vi "ChoosePass.vi"(6 "OffensivePlay":T1, 8 "error in (no error)":errorcluster, 9 "Stk/2ndStk":enum16{"Striker", "2ndStriker"}(ring), 10 "Game":refnum<class "Game.lvclass">, 11 "Play in":refnum<class "Play.lvclass">) -> (0 "error out":errorcluster, 2 "Factor Pass":dbl, 3 "Play out":refnum<class "Play.lvclass">)   [LabVIEW 2023, in "Play.lvclass"]
uses:
  Play.lvclass
  Game_class/Game.lvclass
  Team_class/OffensivePlay.ctl
  Robot_class/roles.ctl
  Utilities_class/Utilities.lvclass
  Game_class/Game.lvclass/Game.ctl
  Team_class/Team.lvclass/Team.ctl
  Object_class/Object.lvclass/Object.ctl
  Robot_class/Robot.lvclass/Robot.ctl
  Referee_class/Referee.lvclass/Referee.ctl
  Object_class/Read x.vi
  Object_class/Read y.vi
  Robot_class/Read role.vi
  Robot_class/Read id.vi
  68f59049-f2ff-4715-8400-83112da4dd7c.vi
  Referee_class/Read enemy_goalie_id.vi
  Team_class/Read RobotRef.vi
  Game_class/Read OffensiveTeam.vi
  Game_class/Read BallRef.vi
  Game_class/Read FieldRef.vi
  Game_class/Read EnemyRef.vi
  Game_class/Read Referee.vi
  <vilib>/Array/Sort 2D Array - Pop Stack.vi
  <vilib>/Array/Sort 2D Array - Push Stack.vi
  68f59049-f2ff-4715-8400-83112da4dd7c.vi/269d4b3b-47f5-49e3-8884-44851e4dd9d5.vi
  68f59049-f2ff-4715-8400-83112da4dd7c.vi/6d99389c-673d-4efb-bf33-19b32bcf4cf8.vi
  Ally_class/Ally.lvclass
  C:/Users/roboi/Downloads/VSS_AI-Larc2023/Team_class/Team.lvclass
  Robot_class/Robot.lvclass
  C:/Users/roboi/Downloads/VSS_AI-Larc2023/Object_class/Object.lvclass
  Enemy_class/Enemy.lvclass
  Ball_class/Ball.lvclass
  Field_class/Field.lvclass
  Referee_class/Referee.lvclass
panel:
  in  "y":dbl=0.2
  in  "y2":dbl=0.17
  in  "y3":dbl=0.4
  in  "y4":dbl=0.16
  in  "y5":dbl=0.07
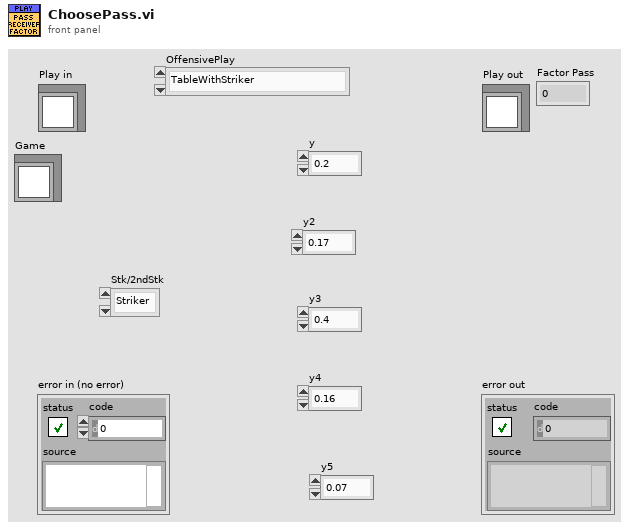
[diagram p1: front panel]
types:
  T1 = typedef "OffensivePlay.ctl" = enum16{"TableWithStriker", "TableWith2ndStrikerPlay", "PrepareDoublePass", "PrepareRollToPass", "SimplePass", "PreparePass", "PassToStriker", "BallOutOfField", "PassTo2ndStriker", "StopOffensive", "Prepare Penalty Enemy", "EnemyPossessionAtEnemyField", "EnemyPossesionAtOurField", "TestPlay", "PreparePenaltyAlly", "KickPenaltyAlly", "PrepareKickoffAlly", "PrepareKickoffEnemy", "IndirectEnemy", "DirectEnemy", "NormalGame", "DirectKick", "Pass", "Halt", "Timeout", "PassPlay", "PenaltyEnemy"}
  T2 = typedef "roles.ctl" = enum16{"BallChallengerAttackerVSS", "NormalAttackerVSS", "AttackerAimGoalVSS", "DefenderAreaVSS", "KeeperVSS", "Tabler", "TableFinalizer", "PrepareRollToPassRoller", "PrepareRollToPassReceiver", "SimplePassRoll", "SimplePassRollReceiver", "PenaltyDefense", "PreparePassReceiver 2", "PreparePassReceiver 1", "PassObserver", "Timeout", "Goto", "ZigZag", "None", "BallOutOfField", "DefenderArea", "Duelist", "AttackerStop", "FollowAttacker", "KeeperRole", "KickPenalty", "AttackerAimGoal", "AttackerBlock", "Marker", "Halt", "Shoot", "PassKicker", "PassReceiver", "TestRole", "PenaltyAttacker"}
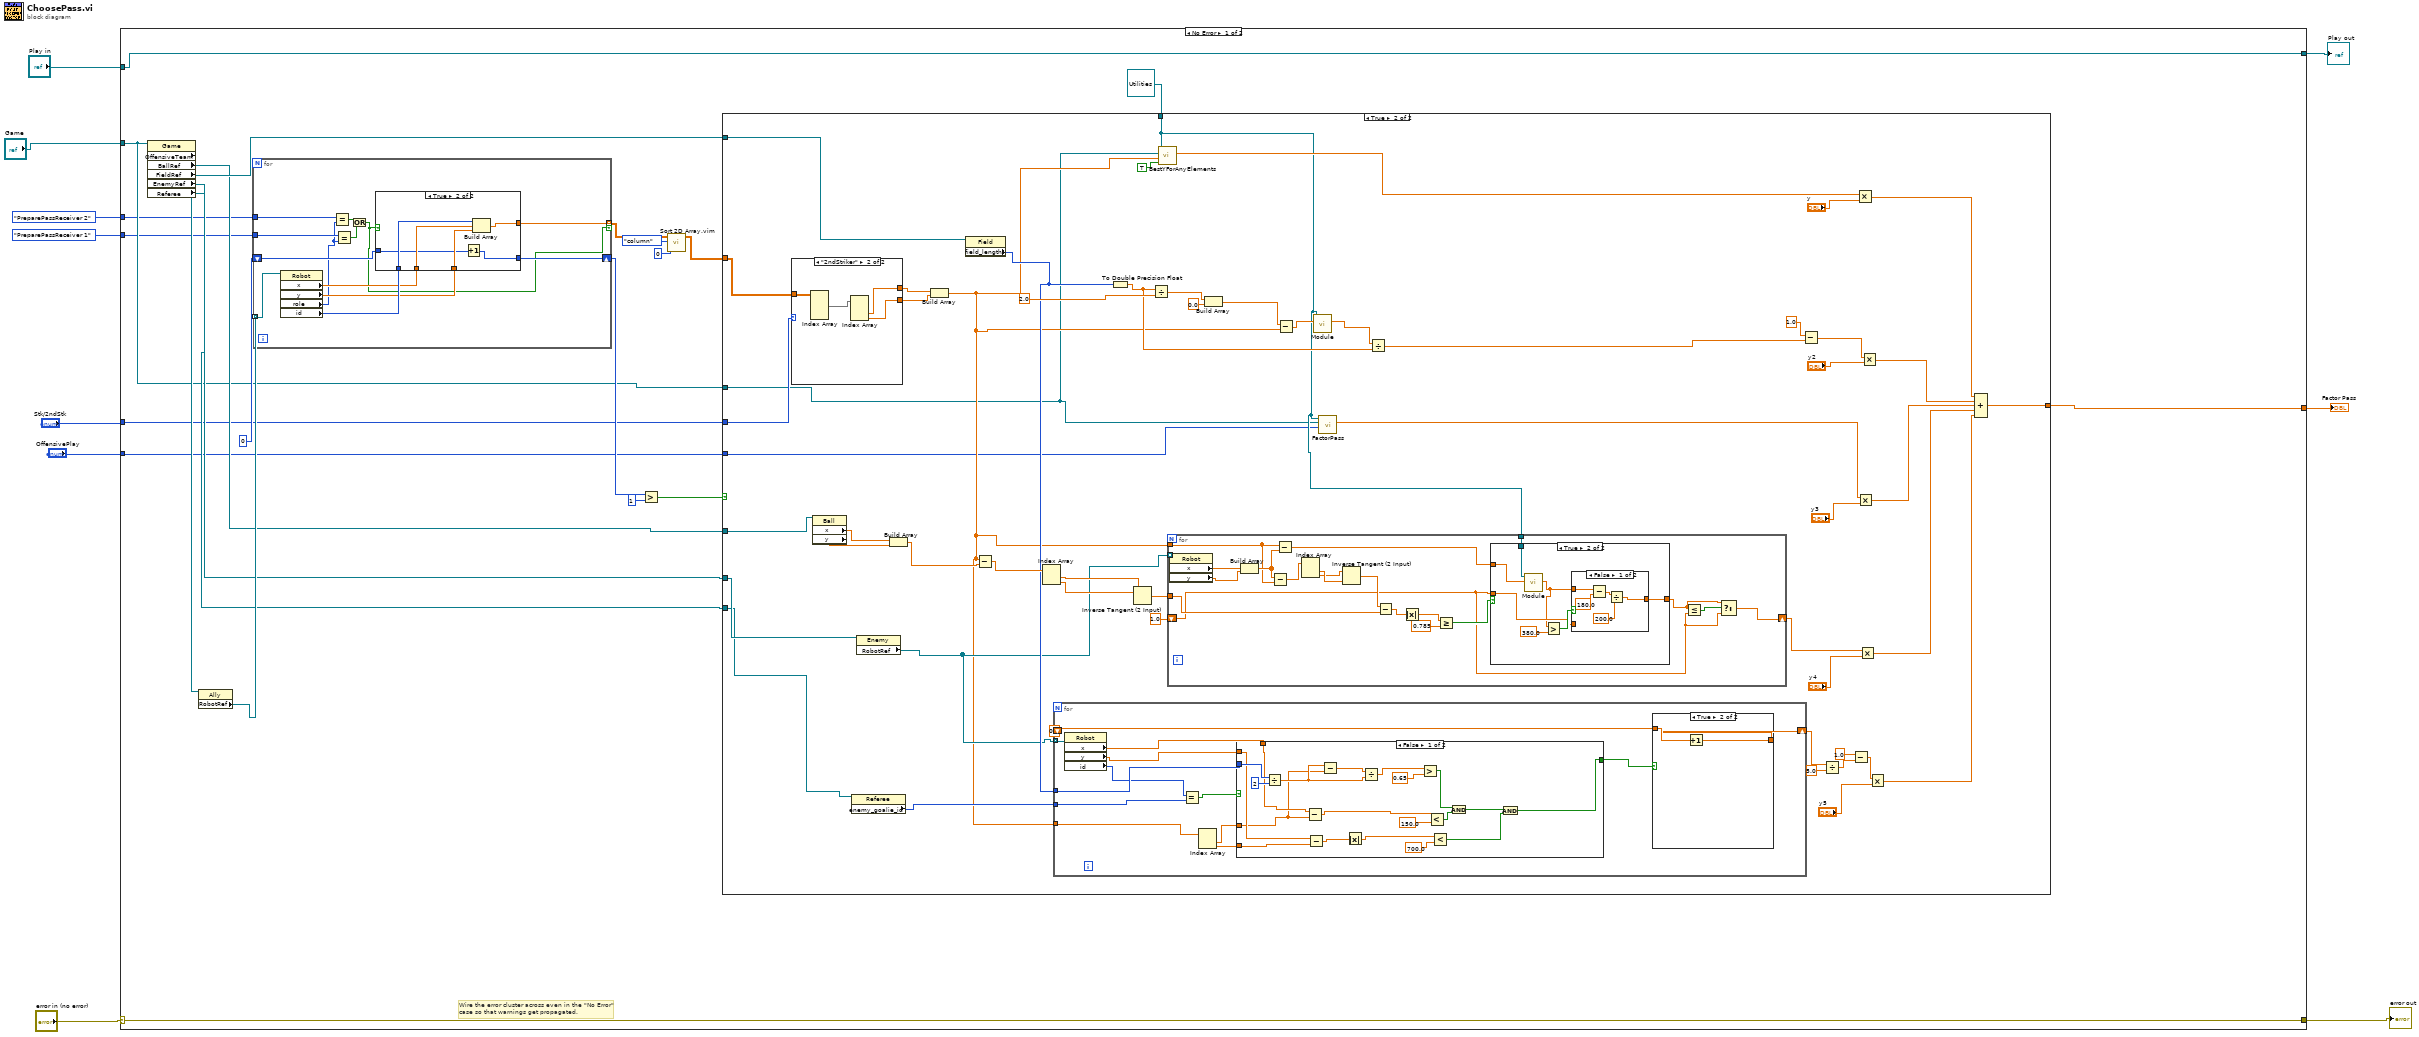
[diagram p0: block diagram]
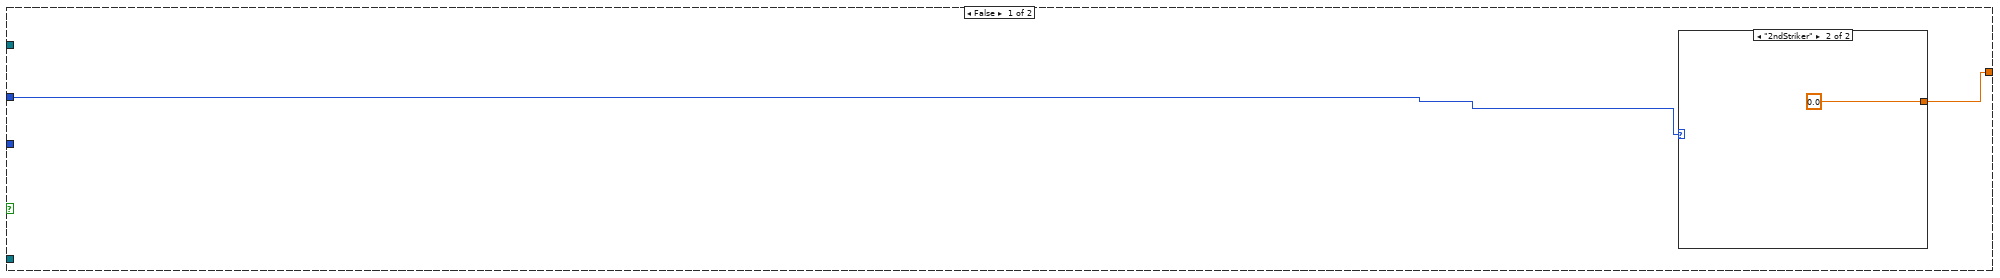
[diagram p2: hidden frame]
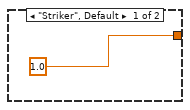
[diagram p3: hidden frame]
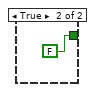
[diagram p4: hidden frame]
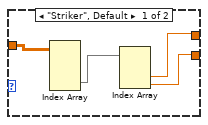
[diagram p8: hidden frame]
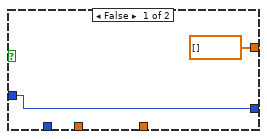
[diagram p9: hidden frame]
diagram:
  n1 = case shown="No Error" "error in (no error)" {
    selector: "error in (no error)" -> [w33 w192]
    tunnel: [w33 w192] -> w5
    tunnel: [w18 _] -> w8
    tunnel: "Play in" -> [w17 _]
    tunnel: [w17 _] -> w9
    tunnel: "Game" -> [w16 _]
    tunnel: "Stk/2ndStk" -> [w14 _]
    tunnel: roles."PreparePassReceiver 1" ("role") -> [w13 _]
    tunnel: roles."PreparePassReceiver 2" ("role") -> [w12 _]
    tunnel: "OffensivePlay" -> [w11 _]
    frame No Error {
      # "Wire the error cluster across even in the \"No Error\"\ncase so that warnings get propagated."
      n2 = property class="Game"(reference=w16) -> ("OffensiveTeam"=w32:refnum<class "Ally.lvclass">, "BallRef"=w21:refnum<class "Ball.lvclass">, "FieldRef"=w22:refnum<class "Field.lvclass">, "EnemyRef"=w20:refnum<class "Enemy.lvclass">, "Referee"=w19:refnum<class "Referee.lvclass">)  [unwired: 1 in, 2 out]
      n3 = property class="Ally"(reference=w32) -> ("RobotRef"=w31:refnum<class "Robot.lvclass">[])  [unwired: 1 in, 2 out]
      n4 = for {
        tunnel: w31 -> [w183] mode=indexing
        shift-right: [w178] -> w26
        shift-left: 0 -> [w179]
        tunnel: [w177] -> w29 mode=indexing if=w171
        tunnel: w13 -> [w176]
        tunnel: w12 -> [w174]
        n5 = property class="Robot"(reference=w183) -> ("x"=w181:dbl, "y"=w180:dbl, "role"=w173:T2, "id"=w182:i32)  [unwired: 1 in, 2 out]
        n6 = Equal?(x=w174, y=w173) -> (x = y?=w175:bool)
        n7 = Equal?(x=w176, y=w173) -> (x = y?=w172:bool)
        n8 = Or(x=w175, y=w172) -> (x .or. y?=w171:bool)
        n9 = case shown="True" w171 {
          tunnel: w182 -> [_ w189]
          tunnel: w181 -> [_ w191]
          tunnel: w180 -> [_ w190]
          tunnel: w179 -> [w184 w188]
          tunnel: [w184 w187] -> w178
          tunnel: [dbl[] [] w186] -> w177
          frame False {
          }
          frame True {
            n10 = Increment(x=w188) -> (x+1=w187:i32)
            n11 = Build Array(w189, w191, w190) -> (w186:dbl[])
          }
        }
      }
      n12 = Greater?(x=w26, y=1) -> (0:w24:bool)
      n13 = call "Sort 2D Array.vim"("index"=0, "dimension to index (column)"=enum16{"column", "row"}."column", "2D array"=w29) -> ("sorted 2D array"=w23:dbl[][])  [unwired: 7 in, 1 out]
      n14 = case shown="True" w24 {
        tunnel: w23 -> [_ w91]
        tunnel: w22 -> [_ w52]
        tunnel: w21 -> [_ w72]
        tunnel: w20 -> [_ w64]
        tunnel: w19 -> [_ w45]
        tunnel: [w35 w53] -> w18
        tunnel: w16 -> [_ w39]
        tunnel: refnum<class "Utilities.lvclass"> refnum ("Utilities in") -> [_ w43]
        tunnel: w14 -> [w34 w44]
        tunnel: w11 -> [_ w38]
        frame False {
          n15 = case shown="\"2ndStriker\"" w34 {
            tunnel: [1.0 0.0] -> w35
            frame "Striker", Default {
            }
            frame "2ndStriker" {
            }
          }
        }
        frame True {
          n16 = case shown="\"2ndStriker\"" w44 {
            tunnel: w91 -> [w166 w170]
            tunnel: [w164 w168] -> w90
            tunnel: [w163 w167] -> w89
            frame "Striker", Default {
              n17 = Index Array(array=w166) -> (element #2=w165:dbl[])  [unwired: 4 in, 1 out]
              n18 = Index Array(array=w165) -> (element #2=w164:dbl, element #3=w163:dbl)  [unwired: 3 in, 1 out]
            }
            frame "2ndStriker" {
              n19 = Index Array(array=w170) -> (element #1=w169:dbl[])  [unwired: 4 in, 1 out]
              n20 = Index Array(array=w169) -> (element #2=w168:dbl, element #3=w167:dbl)  [unwired: 3 in, 1 out]
            }
          }
          n21 = property class="Ball"(reference=w72) -> ("x"=w71:dbl, "y"=w70:dbl)  [unwired: 1 in, 2 out]
          n22 = property class="Referee"(reference=w45) -> ("enemy_goalie_id"=w46:i32)  [unwired: 1 in, 2 out]
          n23 = property class="Enemy"(reference=w64) -> ("RobotRef"=w47:refnum<class "Robot.lvclass">[])  [unwired: 1 in, 2 out]
          n24 = Build Array(w71, w70) -> (w69:dbl[])
          n25 = Build Array(w90, w89) -> (w40:dbl[])
          n26 = property class="Field"(reference=w52) -> ("field_length"=w51:i32)  [unwired: 1 in, 2 out]
          n27 = Subtract(x=w40, y=w69) -> (x-y=w68:dbl[])
          n28 = Index Array(array=w68) -> (element #1=w66:dbl, element #2=w67:dbl)  [unwired: 2 in]
          n29 = for {
            tunnel: w40 -> [w98]
            shift-right: [w103] -> w59
            shift-left: 0.0 -> [w104]
            tunnel: w46 -> [w102]
            tunnel: w51 -> [w99]
            tunnel: w47 -> [w95] mode=indexing
            n30 = property class="Robot"(reference=w95) -> ("x"=w94:dbl, "y"=w93:dbl, "id"=w92:i32)  [unwired: 1 in, 2 out]
            n31 = Equal?(x=w92, y=w102) -> (x = y?=w101:bool)
            n32 = Index Array(array=w98) -> (element #1=w97:dbl, element #2=w96:dbl)  [unwired: 2 in]
            n33 = case shown="False" w101 {
              tunnel: [w106 FALSE] -> w100
              tunnel: w99 -> [w124 _]
              tunnel: w94 -> [w117 _]
              tunnel: w97 -> [w105 _]
              tunnel: w93 -> [w115 _]
              tunnel: w96 -> [w114 _]
              frame False {
                n34 = Divide(x=w124, y=u32 2) -> (x/y=w121:dbl)
                n35 = Subtract(x=w117, y=w105) -> (x-y=w116:dbl)
                n36 = Subtract(x=w115, y=w114) -> (x-y=w113:dbl)
                n37 = Subtract(x=w121, y=w105) -> (x-y=w122:dbl)
                n38 = Absolute Value(x=w113) -> (abs(x)=w112:dbl)
                n39 = Divide(x=w122, y=w121) -> (x/y=w120:dbl)
                n40 = Greater?(x=w120, y=0.65) -> (0:w110:bool)
                n41 = Less?(x=w116, y=150.0) -> (x < y?=w109:bool)
                n42 = Less?(x=w112, y=700.0) -> (x < y?=w107:bool)
                n43 = And(x=w110, y=w109) -> (x .and. y?=w108:bool)
                n44 = And(x=w108, y=w107) -> (x .and. y?=w106:bool)
              }
              frame True {
              }
            }
            n45 = case shown="True" w100 {
              tunnel: w104 -> [w126 w128]
              tunnel: [w126 w127] -> w103
              frame False {
              }
              frame True {
                n46 = Increment(x=w128) -> (x+1=w127:dbl)
              }
            }
          }
          n47 = To Double Precision Float(number=w51) -> (double precision float=w82:dbl)
          n48 = Inverse Tangent (2 Input)(1:w66, 2:w67) -> (0:w65:dbl)
          n49 = Divide(x=w82, y=2.0) -> (x/y=w87:dbl)
          n50 = call "BestYForAnyElements.vi"("inimigos"=TRUE, "Position to be analyzed"=w40, "Game"=w39, "Utilities in"=w43) -> ("Goal Gap"=w48:dbl)  [unwired: 6 in, 1 out]
          n51 = for {
            tunnel: w65 -> [w143]
            tunnel: w40 -> [w133]
            shift-right: [w135] -> w63
            shift-left: 1.0 ("element") -> [w134]
            tunnel: w47 -> [w132] mode=indexing
            tunnel: w43 -> [w129]
            n52 = property class="Robot"(reference=w132) -> ("x"=w131:dbl, "y"=w130:dbl)  [unwired: 1 in, 2 out]
            n53 = Build Array(w131, w130) -> (w139:dbl[])
            n54 = Subtract(x=w139, y=w133) -> (x-y=w148:dbl[])
            n55 = Subtract(x=w133, y=w139) -> (x-y=w138:dbl[])
            n56 = Index Array(array=w148) -> (element #1=w145:dbl, element #2=w144:dbl)  [unwired: 2 in]
            n57 = Inverse Tangent (2 Input)(1:w145, 2:w144) -> (0:w147:dbl)
            n58 = Subtract(x=w147, y=w143) -> (x-y=w146:dbl)
            n59 = Absolute Value(x=w146) -> (abs(x)=w141:dbl)
            n60 = Greater Or Equal?(x=w141, y=0.785) -> (x >= y?=w140:bool)
            n61 = case shown="True" w140 {
              tunnel: w134 -> [w149 w153]
              tunnel: w138 -> [_ w152]
              tunnel: [w149 w155] -> w136
              tunnel: w129 -> [_ w151]
              frame False {
              }
              frame True {
                n62 = call-dynamic "Module.vi"("2D vector"=w152, "Utilities in"=w151) -> ("Modulo"=w150:dbl)  [unwired: 7 in, 2 out]
                n63 = Greater?(x=w150, y=380.0) -> (0:w154:bool)
                n64 = case shown="False" w154 {
                  tunnel: w153 -> [_ w162]
                  tunnel: [w161 w162] -> w155
                  tunnel: w150 -> [w157 _]
                  frame False {
                    n65 = Subtract(x=w157, y=180.0) -> (x-y=w159:dbl)
                    n66 = Divide(x=w159, y=200.0) -> (x/y=w161:dbl)
                  }
                  frame True {
                  }
                }
              }
            }
            n67 = Less Or Equal?(x=w136, y=w134) -> (x <= y?=w137:bool)
            n68 = Select(t=w136, s=w137, f=w134) -> (s? t:f=w135:dbl)
          }
          n69 = Build Array(w87, 0.0 ("element")) -> (w85:dbl[])
          n70 = Subtract(x=w85, y=w40) -> (x-y=w50:dbl[])
          n71 = call-dynamic "Module.vi"("2D vector"=w50, "Utilities in"=w43) -> ("Modulo"=w49:dbl)  [unwired: 7 in, 2 out]
          n72 = call-dynamic "FactorPass.vi"("OffensivePlay"=w38, "Game"=w39, "Utilities in"=w43) -> ("Critério de marcação Normalizado"=w42:dbl)  [unwired: 6 in, 2 out]
          n73 = Divide(x=w49, y=w82) -> (x/y=w84:dbl)
          n74 = Subtract(x=1.0, y=w84) -> (x-y=w81:dbl)
          n75 = Divide(x=w59, y=5.0) -> (x/y=w57:dbl)
          n76 = Subtract(x=1.0, y=w57) -> (x-y=w55:dbl)
          n77 = Multiply(x=w48, y="y") -> (x*y=w79:dbl)
          n78 = Multiply(x=w42, y="y3") -> (x*y=w76:dbl)
          n79 = Multiply(x=w63, y="y4") -> (x*y=w75:dbl)
          n80 = Multiply(x=w81, y="y2") -> (x*y=w80:dbl)
          n81 = Multiply(x=w55, y="y5") -> (x*y=w60:dbl)
          n82 = Compound Arithmetic op=ADD(w79, w80, w76, w75, w60) -> (w53:dbl)
        }
      }
    }
    frame Error {
    }
  }
  "error out" <- w5
  "Play out" <- w9
  "Factor Pass" <- w8
